vi "Recursive Folder List_lvcicd.vi"(4 "Folders to Exclude":string[](array[string])=[".git"], 6 "pattern":string="_warehouse", 8 "error in (no error)":errorcluster, 9 "Continue Recursing on Error? (F)":bool, 11 "Folder Path":path=path "D:/OneDrive - NI/Prototype/SIL/engine") -> (0 "error out":errorcluster, 1 "Number of Folders":i32=1, 2 "All Folders":path[](array[path])=[path "D:/OneDrive - NI/Prototype/SIL/engine/_warehouse"], 3 "dup Folder Path":path=path "D:/OneDrive - NI/Prototype/SIL/engine")   [LabVIEW 2014]
doc: "Lists the contents of a folder or LLB."
uses:
  <userlib>/_OpenG.lib/file/file.llb/Build Path - File Names Array__ogtk.vi
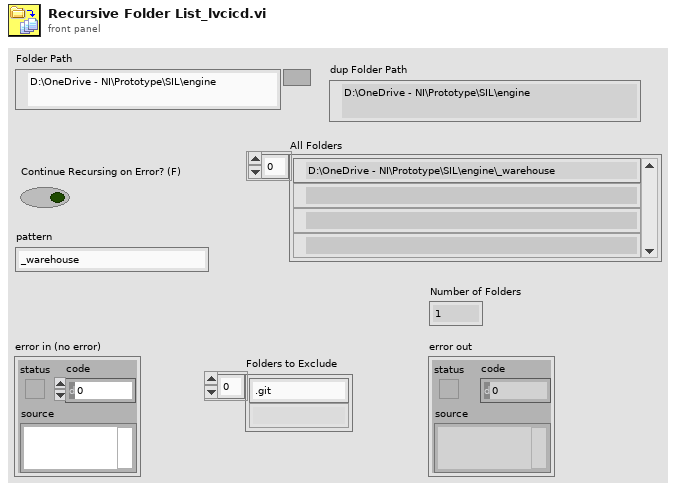
[diagram p1: front panel]
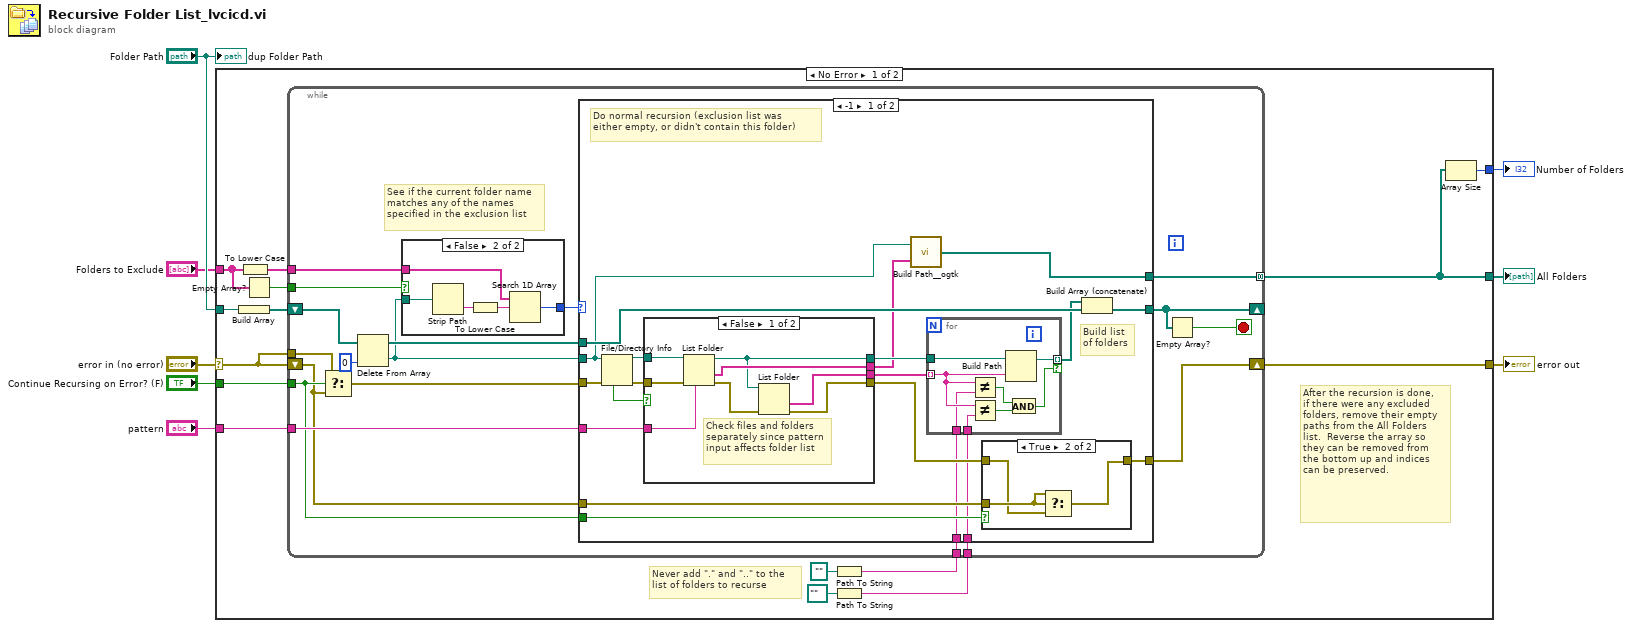
[diagram p0: block diagram]
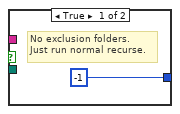
[diagram p2: hidden frame]
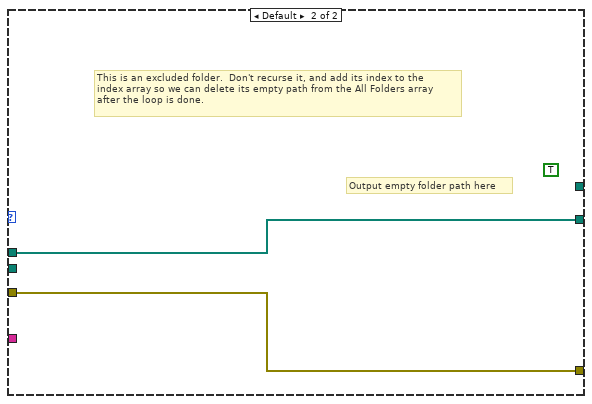
[diagram p5: hidden frame]
diagram:
  n1 = case shown="No Error" "error in (no error)" {
    selector: "error in (no error)" -> [w17 w91]
    tunnel: "Folder Path" -> [w23 _]
    tunnel: [w19 _] -> w8
    tunnel: [w20 w91] -> w7
    tunnel: [w9 _] -> w5
    tunnel: "pattern" -> [w21 _]
    tunnel: "Continue Recursing on Error? (F)" -> [w18 _]
    tunnel: "Folders to Exclude" -> [w15 _]
    frame No Error {
      # "Never add \".\" and \"..\" to the list of folders to recurse"
      # "After the recursion is done,\nif there were any excluded\nfolders, remove their empty\npaths from the All Folders\nlist.  Reverse the array so\nthey can be removed from\nthe bottom up and indices\ncan be preserved."
      n2 = Build Array(w23) -> (w22:path[])
      n3 = To Lower Case(string=w15) -> (all lower case string=w16:string[])
      n4 = Empty Array?(array=w15) -> (empty?=w14:bool)
      n5 = Path To String(path=path "") -> (string=w11:string)
      n6 = Path To String(path=path "..") -> (string=w10:string)
      n7 = while {
        shift-left: w22 -> [w41]
        shift-right: [w39] -> _
        shift-right: [w33] -> w20
        shift-left: w17 -> [w32]
        tunnel: [w30] -> w9 mode=concatenating
        tunnel: w21 -> [w40]
        tunnel: w18 -> [w34]
        tunnel: w17 -> [w35]
        tunnel: w16 -> [w28]
        tunnel: w14 -> [w29]
        tunnel: w11 -> [w25]
        tunnel: w10 -> [w24]
        stop <- w38 stop-if-true
        # "See if the current folder name\nmatches any of the names\nspecified in the exclusion list"
        n8 = Select(t=w35, s=w34, f=w32) -> (s? t:f=w36:errorcluster)
        n9 = Delete From Array(array=w41, index=0) -> (deleted portion=w27:path, array with subset deleted=w31:path[])  [unwired: 1 in]
        n10 = case shown="False" w29 {
          tunnel: w28 -> [_ w44]
          tunnel: w27 -> [_ w47]
          tunnel: [-1 ("index of element") w43] -> w26
          frame True {
            # "No exclusion folders.\nJust run normal recurse."
          }
          frame False {
            n11 = Strip Path(path=w47) -> (name=w46:string)  [unwired: 1 out]
            n12 = To Lower Case(string=w46) -> (all lower case string=w45:string)
            n13 = Search 1D Array(1D array=w44, element=w45) -> (index of element=w43:i32)  [unwired: 1 out]
          }
        }
        n14 = case shown="-1" w26 {
          tunnel: w40 -> [w65 _]
          tunnel: [w63 w90] -> w39
          tunnel: w27 -> [w50 _]
          tunnel: w36 -> [w59 w89]
          tunnel: w34 -> [w57 _]
          tunnel: [w56 w89] -> w33
          tunnel: w32 -> [w55 _]
          tunnel: w31 -> [w54 w90]
          tunnel: [w48 _] -> w30
          tunnel: w25 -> [w52 _]
          tunnel: w24 -> [w51 _]
          frame -1 {
            # "Build list\nof folders"
            # "Do normal recursion (exclusion list was\neither empty, or didn't contain this folder)"
            n15 = File/Directory Info(path=w50, error in=w59) -> (path out=w61:path, error out=w62:errorcluster, shortcut=w60:bool)  [unwired: 4 out]
            n16 = case shown="False" w60 {
              tunnel: [w82 _] -> w49
              tunnel: [w81 w84] -> w66
              tunnel: [w80 w83] -> w58
              tunnel: w65 -> [w79 _]
              tunnel: [w75 _] -> w64
              tunnel: w62 -> [w78 w83]
              tunnel: w61 -> [w77 w84]
              frame False {
                # "Check files and folders\nseparately since pattern\ninput affects folder list"
                n17 = List Folder(path=w77, pattern=w79, error in=w78) -> (path out=w81:path, folder names=w82:string[], error out=w76:errorcluster)  [unwired: 2 out]
                n18 = List Folder(path=w81, error in=w76) -> (folder names=w75:string[], error out=w80:errorcluster)  [unwired: 4 out]
              }
              frame True {
                # "Do not attempt to recurse the contents of folder shortcuts"
              }
            }
            n19 = call-poly <userlib>:"Build Path__ogtk.vi"("name or relative path"=w49, "base path"=w50) -> ("appended path"=w48:path[])
            n20 = for {
              tunnel: w66 -> [w74]
              tunnel: [w73] -> w53 mode=indexing if=w72
              tunnel: w64 -> [w71] mode=indexing
              tunnel: w52 -> [w70]
              tunnel: w51 -> [w69]
              n21 = Not Equal?(x=w71, y=w70) -> (x != y?=w67:bool)
              n22 = Not Equal?(x=w71, y=w69) -> (x != y?=w68:bool)
              n23 = Build Path(base path=w74, name or relative path=w71) -> (appended path=w73:path)
              n24 = And(x=w67, y=w68) -> (x .and. y?=w72:bool)
            }
            n25 = case shown="True" w57 {
              tunnel: w58 -> [w85 w87]
              tunnel: [w85 w86] -> w56
              tunnel: w55 -> [_ w88]
              frame False {
              }
              frame True {
                n26 = Select(t=w88, s=w88, f=w87) -> (s? t:f=w86:errorcluster)
              }
            }
            n27 = Build Array (concatenate)(w53, w54) -> (w63:path[])
          }
          frame Default {
            (unwired) TRUE
            # "Output empty folder path here"
            # "This is an excluded folder.  Don't recurse it, and add its index to the\nindex array so we can delete its empty path from the All Folders array\nafter the loop is done."
          }
        }
        n28 = Empty Array?(array=w39) -> (empty?=w38:bool)
      }
      n29 = Array Size(array=w9) -> (size(s)=w19:i32)
    }
    frame Error {
    }
  }
  "Number of Folders" <- w8
  "error out" <- w7
  "All Folders" <- w5
  "dup Folder Path" <- "Folder Path"
